vi "Example_EdgeConfig.vi"() -> ()   [LabVIEW 2013]
panel:
  in  "edge":enum32{"Rising Edge", "Falling Edge"}(ring)
  in  "nSlot":i32=5
  in  "nChassis":i32=1
  in  "partNumber":string="SD-PXE-TDC-H0002"
  out "countRate":i32
  in  "stop":bool
  in  "nChannel":i32
  out "errorOut":errorcluster
  # "Module Under Test"
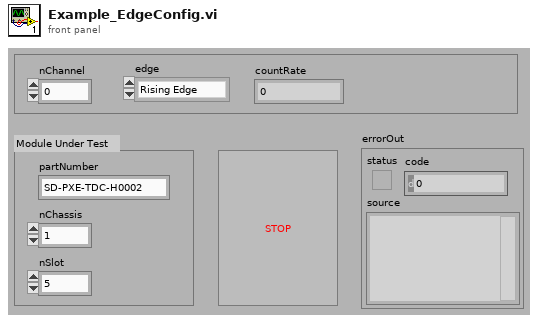
[diagram p1: front panel]
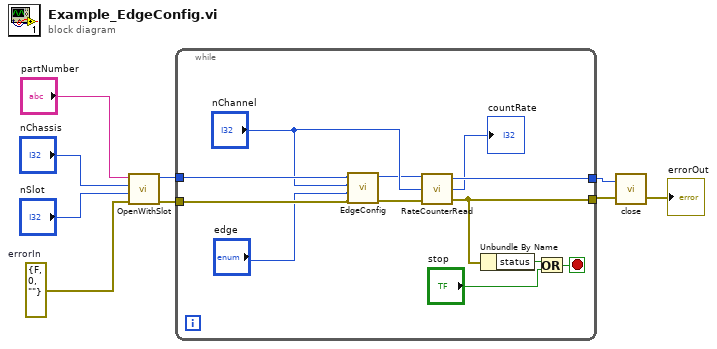
[diagram p0: block diagram]
diagram:
  w9 = errorcluster {"status"=FALSE, "code"=0, "source"=""}  # errorIn
  n1 = call <vilib>:"OpenWithSlot.vi"("errorIn"=w9, "nSlot"="nSlot", "nChassis"="nChassis", "partNumber"="partNumber") -> ("errorOut"=w5:errorcluster, "moduleID"=w4:i32)  [unwired: 2 in]
  n2 = while {
    tunnel: w5 -> [w15]
    tunnel: [w12] -> w3
    tunnel: w4 -> [w19]
    tunnel: [w21] -> w2
    stop <- w13 stop-if-true
    n3 = call <vilib>:"EdgeConfig.vi"("errorIn"=w15, "edge"="edge", "nChannel"="nChannel", "moduleID"=w19) -> ("errorOut"=w16:errorcluster, "moduleIDout"=w17:i32)  [unwired: 2 in]
    n4 = call <vilib>:"RateCounterRead.vi"("errorIn"=w16, "nChannel"="nChannel", "moduleID"=w17) -> ("errorOut"=w12:errorcluster, "countRate"=→"countRate":i32, "moduleIDout"=w21:i32)
    n5 = Unbundle By Name(w12) -> ("status"=w11:bool)
    n6 = Or(x=w11, y="stop") -> (x .or. y?=w13:bool)
  }
  n7 = call <vilib>:"close.vi"("errorIn"=w3, "moduleID"=w2) -> ("errorOut"=→"errorOut":errorcluster)  [unwired: 1 in]
